vi "Lesson 2-1 Collecting a larger sample size.vi"() -> ()   [LabVIEW 2020]
uses:
  aqn/HRM-AQN-input_clust.ctl
panel:
  in  "samples [s]":i32
  out "Raw collected data":waveform(dbl)(graph)
  out "error out":errorcluster
  in  "stop":bool
  out "Raw data":waveform(dbl)(graph)
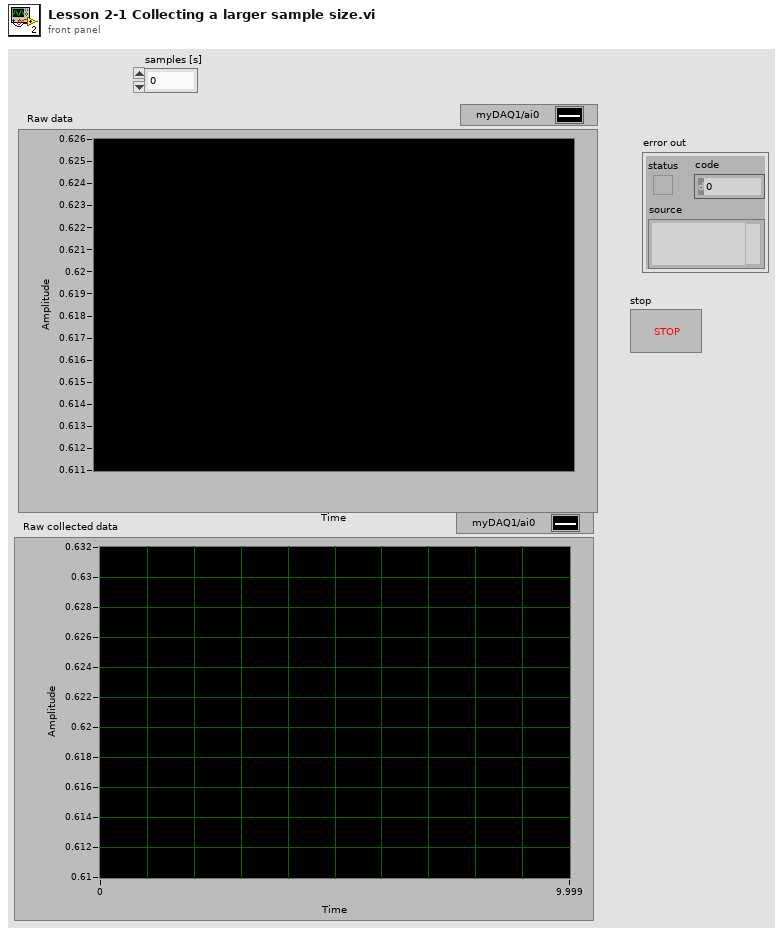
[diagram p1: front panel]
types:
  T1 = typedef "HRM-AQN-input_clust.ctl" = cluster{"physical channels":tag, "myDAQ task":refnum<k21>}
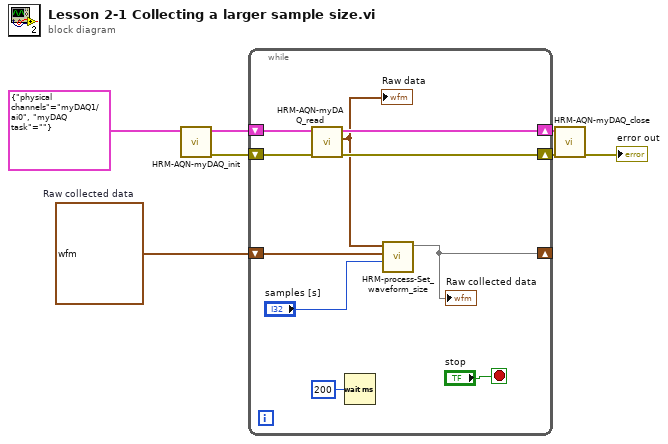
[diagram p0: block diagram]
diagram:
  w1 = waveform(dbl) {"t0"=timestamp(0 s since 1904-01-01), "dt"=1.0, "Y"=[]}  # Raw collected data
  n1 = call "HRM-AQN-myDAQ_init.vi"("AQN cluster in"=T1 {"physical channels"="myDAQ1/ai0", "myDAQ task"=""}) -> ("error out"=w7:errorcluster, "AQN cluster out"=w3:T1)  [unwired: 9 in]
  n2 = while {
    shift-right: [w12] -> w2
    shift-left: w3 -> [w13]
    shift-right: [w16] -> w6
    shift-left: w7 -> [w17]
    shift-right: [w9] -> _
    shift-left: w1 -> [w11]
    stop <- "stop" stop-if-true
    n3 = call "HRM-AQN-myDAQ_read.vi"("error in (no error)"=w17, "AQN cluster in"=w13) -> ("error out"=w16:errorcluster, "data"=w10:waveform(dbl), "AQN cluster out"=w12:T1)  [unwired: 7 in]
    "Raw data" <- w10
    n4 = Wait (ms)(milliseconds to wait=u32 200) -> ()  [unwired: 1 out]
    n5 = call "HRM-process-Set_waveform_size.vi"("samples [s]"="samples [s]", "Raw collected data"=w11, "Raw data in"=w10) -> (3:w9)  [unwired: 7 in, 1 out]
    "Raw collected data" <- w9
  }
  n6 = call "HRM-AQN-myDAQ_close.vi"("error in (no error)"=w6, "AQN cluster in"=w2) -> ("error out"=→"error out":errorcluster)  [unwired: 9 in]
